vi "Manage Configuration File.vi"(8 "SAVE MODE":enum16{"DO NOT SAVE", "SAVE .CNF FILE"}(ring), 9 "PROCESSING MODE":enum16{"NONE", "READ", "CREATE"}(ring), 11 "CONFIGURATION CLUSTER":T1) -> (3 "CONFIGURATION CLUSTER OUT":T1)   [LabVIEW 2021]
doc: "Create, read and save the configuration\nfile. Configuration file determines the \nsettings of the AVS-47B and TS-530A, and the VISA resource to be used."
uses:
  <vilib>/Utility/error.llb/DialogType.ctl
panel:
  out "INFO STRING OUT":string
  in  "SENSOR dR/dT":u8(ring) items=["NEGATIVE", "POSITIVE"]
  in  "INTERVAL":u8(ring) items=["NO TS-530A", "1 s", "15 s", "30 s", "45 s", "60 s", "120 s", "240 s", "480 s"]
  in  "HEATER RESISTANCE":dbl=100.0 min=0.0 max=1000.0 format="%_3f"
  in  "SET POINT 2":dbl format="%^_6e"
  in  "PICOBUS ADDRESS":u8=1 min=1 max=15 step=1
  in  "INFO STRING":string
  in  "POWER RANGE":u8(ring) items=["OFF", "1uW", "10uW", "100uW", "1mW", "10mW", "100mW", "1W", ""]
  in  "POWER BIAS":u8(ring) items=["0", "20%", "40%", "60%", "80%", "100%", ""]
  in  "DERIV":u8(ring) items=["0", "1s", "2s", "5s", "10s", "20s", "50s", "100", ""]
  in  "INTG":u8(ring) items=["PD", "2s", "5s", "10s", "20s", "50s", "100s", "200s", "500s", "1000", "LATCHED", "PD", "N/A", "N/A", "N/A", "SHORTED", ""]
  in  "PROP GAIN":u8(ring) items=["5dB", "10dB", "15dB", "20dB", "25dB", "30dB", "35dB", "40dB", "45dB", "50dB", "55dB", "60dB", ""]
  in  "DISABLE AL":u8(ring) items=["ENABLED", "DISABLED"]
  in  "REMOTE":u8(ring) items=["NO", "YES"]
  in  "DIGITAL REFERENCE":u16 max=19999 step=1
  in  "DISPLAY":u8(ring) items=["R", "DR", "ADJ REF", "REFERENCE", "EXC VOLT", "530A HEAT V", "530A HEAT I", "530A SET PT"]
  in  "EXCITATION":u8(ring)=1 items=["NO EXCITATION", "3 uV", "10uV", "30uV", "100uV", "300uV", "1mV", "3mV"]
  in  "RANGE":u8(ring)=7 items=["NO RANGE", "2 Ohms", "20 Ohms", "200 Ohms", "2 kOhms", "20 kOhms", "200 kOhms", "2 MOhms"]
  in  "CHANNEL":u8(ring) items=["CH0", "CH1", "CH2", "CH3", "CH4", "CH5", "CH6", "CH7"]
  in  "INPUT":u8(ring) items=["ZERO", "MEAS", "CAL"]
  in  "VISA RESOURCE":refnum<visa-resource-name>="COM4"
  out "error out":errorcluster
  # "Manage Configuration File.vi"
  # "AVS-47B DEFAULTS"
  # "TS-530A DEFAULTS"
  # "Ohms"
  # "Ohms"
  # "By selecting the Processing Mode and Save Mode suitably, you can:\n- Just save the current configuration file without making any changes\n- Create the configuration cluster from the front panel values and save or not to save it\n- Read the last saved configuration file and output the configuration cluster to be used by other VIs. If reading is unsuccesful, e.g. if the .cnf file is not found, a new file is automatically created from the defaults and a default config cluster is output."
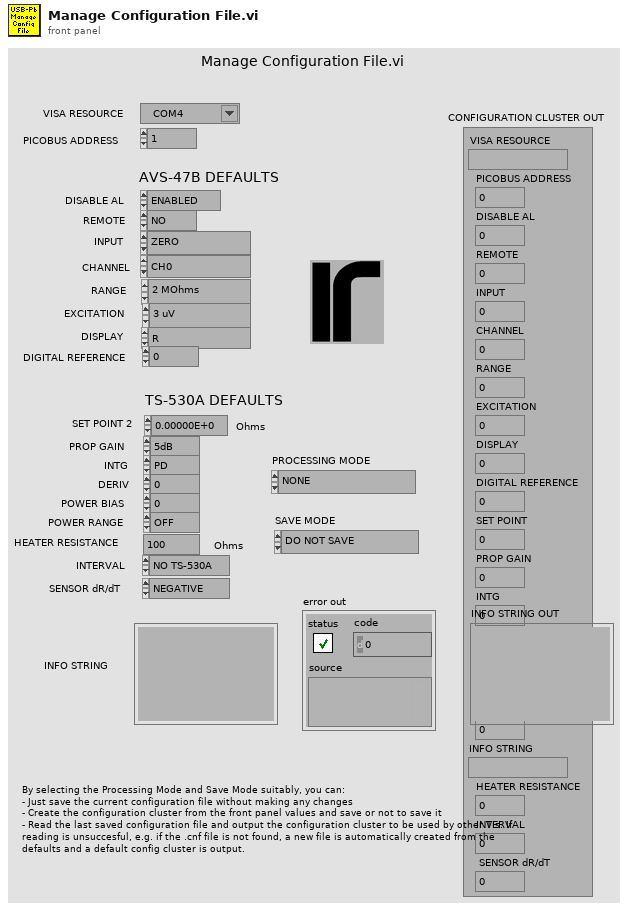
[diagram p1: front panel]
types:
  T1 = cluster{"VISA RESOURCE":refnum<visa-resource-name>, "PICOBUS ADDRESS":u8, "DISABLE AL":u8, "REMOTE":u8, "INPUT":u8, "CHANNEL":u8, "RANGE":u8, "EXCITATION":u8, "DISPLAY":u8, "DIGITAL REFERENCE":u16, "SET POINT":dbl, "PROP GAIN":u8, "INTG":u8, "DERIV":u8, "POWER BIAS":u8, "POWER RANGE":u8, "INFO STRING":string, "HEATER RESISTANCE":dbl, "INTERVAL":u8, " SENSOR dR/dT":u8}
  T2 = cluster{"VISA RESOURCE":refnum<visa-resource-name>, "PICOBUS ADDRESS":u8, "DISABLE AL":u8, "REMOTE":u8, "INPUT":u8, "CHANNEL":u8, "RANGE":u8, "EXCITATION":u8, "DISPLAY":u8, "DIGITAL REFERENCE":u16, "SET POINT 2":dbl, "PROP GAIN":u8, "INTG":u8, "DERIV":u8, "POWER BIAS":u8, "POWER RANGE":u8, "INFO STRING":string, "HEATER RESISTANCE":dbl, "INTERVAL":u8, " SENSOR dR/dT":u8}
  T3 = enum16{"open", "replace", "create", "open or create", "replace or create", "replace or create with confirmation"}
  T4 = typedef "DialogType.ctl" = u16
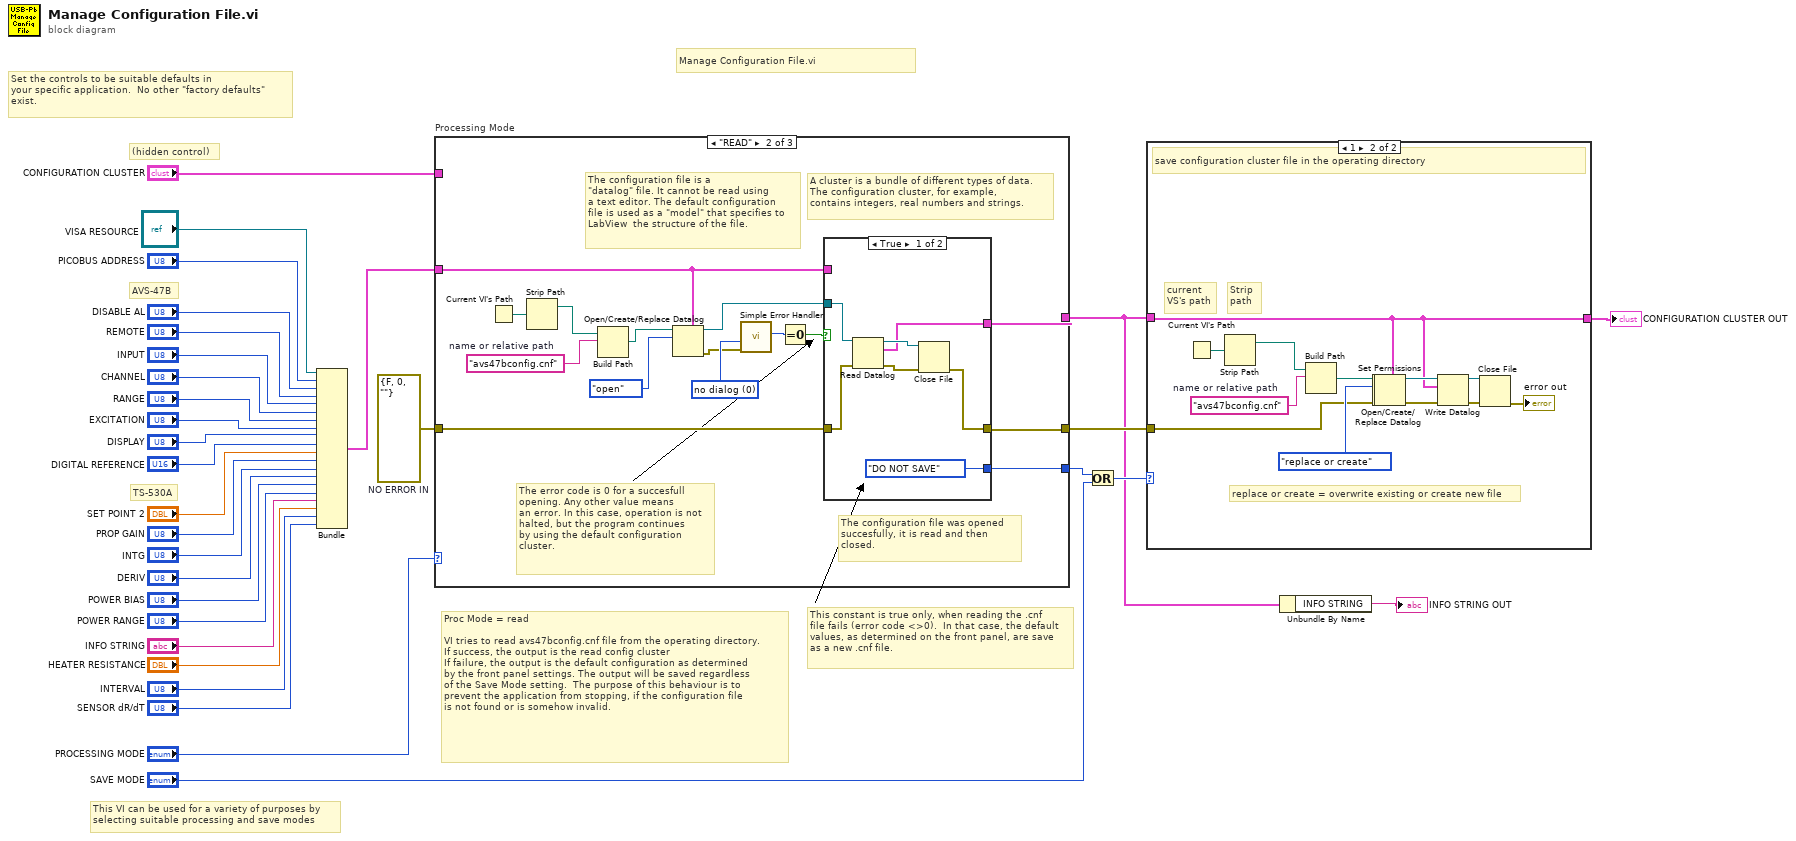
[diagram p0: block diagram]
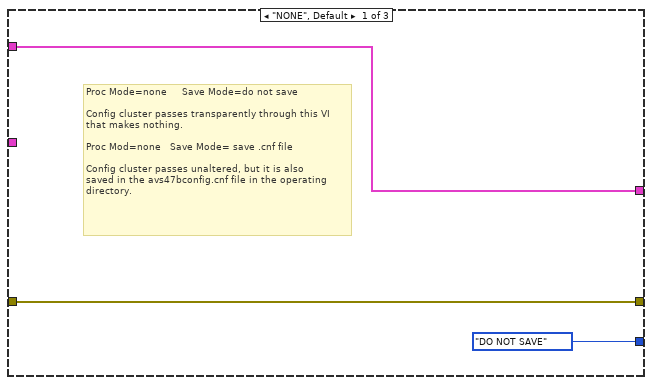
[diagram p3: hidden frame]
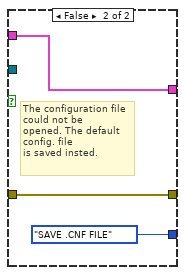
[diagram p4: hidden frame]
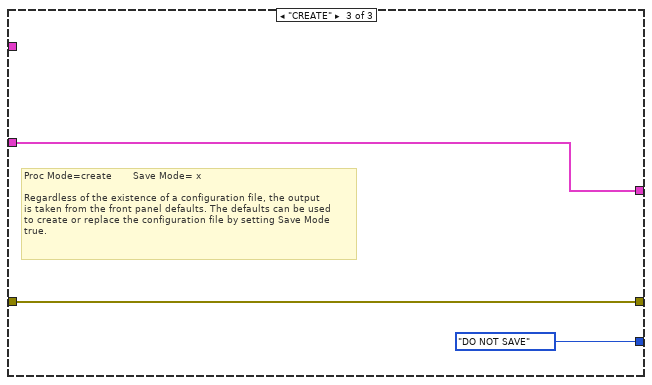
[diagram p5: hidden frame]
diagram:
  w28 = errorcluster {"status"=FALSE, "code"=0, "source"=""}  # NO ERROR IN
  # "Proc Mode = read\n\nVI tries to read avs47bconfig.cnf file from the operating directory.\nIf success, the output is the read config cluster\nIf failure, the output is the default configuration as determined\nby the front panel settings. The output will be saved regardless\nof the Save Mode setting.  The purpose of this behaviour is to\nprevent the application from stopping, if the configuration file\nis not found or is somehow invalid."
  # "Set the controls to be suitable defaults in\nyour specific application.  No other \"factory defaults\"\nexist."
  # "This VI can be used for a variety of purposes by\nselecting suitable processing and save modes"
  # "This constant is true only, when reading the .cnf\nfile fails (error code <>0).  In that case, the default\nvalues, as determined on the front panel, are save\nas a new .cnf file."
  # "Manage Configuration File.vi"
  # "(hidden control)"
  # "TS-530A"
  # "AVS-47B"
  n1 = Bundle("VISA RESOURCE"="VISA RESOURCE", "PICOBUS ADDRESS"="PICOBUS ADDRESS", "DISABLE AL"="DISABLE AL", "REMOTE"="REMOTE", "INPUT"="INPUT", "CHANNEL"="CHANNEL", "RANGE"="RANGE", "EXCITATION"="EXCITATION", "DISPLAY"="DISPLAY", "DIGITAL REFERENCE"="DIGITAL REFERENCE", "SET POINT 2"="SET POINT 2", "PROP GAIN"="PROP GAIN", "INTG"="INTG", "DERIV"="DERIV", "POWER BIAS"="POWER BIAS", "POWER RANGE"="POWER RANGE", "INFO STRING"="INFO STRING", "HEATER RESISTANCE"="HEATER RESISTANCE", "INTERVAL"="INTERVAL", "SENSOR dR/dT"="SENSOR dR/dT") -> (w29:T2)  [unwired: 1 in]
  n2 = case "Processing Mode" shown="\"READ\"" "PROCESSING MODE" {
    tunnel: "CONFIGURATION CLUSTER" -> [w34 _ _]
    tunnel: [w34 w39 w62] -> w2
    tunnel: w29 -> [_ w38 w62]
    tunnel: w28 -> [w33 w36 w61]
    tunnel: [w33 w37 w61] -> w27
    tunnel: [enum16{"DO NOT SAVE", "SAVE .CNF FILE"}."DO NOT SAVE" ("SAVE MODE 2") w35 enum16{"DO NOT SAVE", "SAVE .CNF FILE"}."DO NOT SAVE" ("SAVE MODE 2")] -> w5
    frame "NONE", Default {
      # "Proc Mode=none     Save Mode=do not save\n   \nConfig cluster passes transparently through this VI\nthat makes nothing.\n\nProc Mod=none   Save Mode= save .cnf file\n\nConfig cluster passes unaltered, but it is also\nsaved in the avs47bconfig.cnf file in the operating\ndirectory."
    }
    frame "READ" {
      w46 = T4 0 items=["no dialog", "OK message", "continue or stop message", "OK message + warnings", "continue/stop + warnings"] ("type of dialog (OK msg:1)")
      w40 = "avs47bconfig.cnf"  # name or relative path
      # "The configuration file was opened\nsuccesfully, it is read and then \nclosed."
      # "The configuration file is a \n\"datalog\" file. It cannot be read using\na text editor. The default configuration\nfile is used as a \"model\" that specifies to\nLabView  the structure of the file."
      # "The error code is 0 for a succesfull\nopening. Any other value means\nan error. In this case, operation is not\nhalted, but the program continues\nby using the default configuration\ncluster."
      # "A cluster is a bundle of different types of data.\nThe configuration cluster, for example, \ncontains integers, real numbers and strings."
      n3 = Current VI's Path() -> (path=w41:path)
      n4 = Strip Path(path=w41) -> (stripped path=w42:path)  [unwired: 1 out]
      n5 = Build Path(base path=w42, name or relative path=w40) -> (appended path=w43:path)
      n6 = Open/Create/Replace Datalog(5:w38, 10:T3."open" ("operation (0:open)"), 11:w43) -> (0:w44:errorcluster, 3:w45:refnum<k1>)  [unwired: 3 in, 1 out]
      n7 = call <vilib>:"Simple Error Handler.vi"("type of dialog (OK msg:1)"=w46, "error in (no error)"=w44) -> ("code out"=w48:i32)  [unwired: 3 in, 4 out]
      n8 = Equal To 0?(x=w48) -> (x = 0?=w49:bool)
      n9 = case shown="True" w49 {
        tunnel: w45 -> [w54 _]
        tunnel: w38 -> [_ w57]
        tunnel: [w53 w57] -> w39
        tunnel: [w52 w59] -> w37
        tunnel: w36 -> [w51 w59]
        tunnel: [enum16{"DO NOT SAVE", "SAVE .CNF FILE"}."DO NOT SAVE" ("SAVE MODE 2") enum16{"DO NOT SAVE", "SAVE .CNF FILE"}."SAVE .CNF FILE" ("SAVE MODE 2")] -> w35
        frame True {
          n10 = Read Datalog(4:w51, 7:w54) -> (0:w56:errorcluster, 2:w53:T2, 3:w55:refnum<k1>)  [unwired: 1 in]
          n11 = Close File(refnum=w55, error in=w56) -> (error out=w52:errorcluster)  [unwired: 1 out]
        }
        frame False {
          # "The configuration file could not be\nopened. The default config. file\nis saved insted."
        }
      }
    }
    frame "CREATE" {
      # "Proc Mode=create       Save Mode= x\n\nRegardless of the existence of a configuration file, the output\nis taken from the front panel defaults. The defaults can be used\nto create or replace the configuration file by setting Save Mode\ntrue."
    }
  }
  n12 = Or(x=w5, y="SAVE MODE") -> (x .or. y?=w3:i32)
  n13 = case shown="1" w3 {
    tunnel: [w63 w65] -> w6
    tunnel: w2 -> [w63 w65]
    tunnel: w27 -> [_ w64]
    frame 0, Default {
      # "do not save nor create configuration file"
    }
    frame 1 {
      w71 = "avs47bconfig.cnf"  # name or relative path
      # "Strip\npath"
      # "current\nVS's path"
      # "replace or create = overwrite existing or create new file"
      # "save configuration cluster file in the operating directory"
      n14 = Current VI's Path() -> (path=w73:path)
      n15 = Strip Path(path=w73) -> (stripped path=w74:path)  [unwired: 1 out]
      n16 = Build Path(base path=w74, name or relative path=w71) -> (appended path=w72:path)
      n17 = Open/Create/Replace Datalog(5:w65, 8:w64, 10:T3."replace or create" ("operation (0:open)"), 11:w72) -> (0:w75:errorcluster, 3:w67:refnum<k1>)  [unwired: 2 in, 1 out]
      n18 = Set Permissions(8:w75, 11:w72) -> (0:w68:errorcluster)  [unwired: 3 in, 1 out]
      n19 = Write Datalog(4:w68, 6:w65, 7:w67) -> (0:w70:errorcluster, 3:w69:refnum<k1>)
      n20 = Close File(refnum=w69, error in=w70) -> (error out=→"error out":errorcluster)  [unwired: 1 out]
    }
  }
  "CONFIGURATION CLUSTER OUT" <- w6
  n21 = Unbundle By Name(w2) -> ("INFO STRING"=→"INFO STRING OUT":string)
